vi "aal_Error Code Pool (Polynomial).vi"(1 "error":T1 items=["No Error"=0, "Err - a"=-1, "Err - b"=-2, "Warn - a"=1, "Warn - b"=2]) -> (0 "error code":i32)   [LabVIEW 2017, in "NI_AALPro.lvlib"]
uses:
  <vilib>/Analysis/NI_AALPro.lvlib
  <vilib>/Analysis/aalutilities.llb/aal_Error Code List (Polynomial).ctl
  <vilib>/Analysis/aalutilities.llb/aal_error code offset.ctl
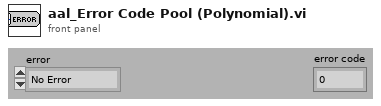
[diagram p1: front panel]
types:
  T1 = typedef "NI_AALPro.lvlib/aal_Error Code List (Polynomial).ctl" = i32
  T2 = typedef "NI_AALPro.lvlib/aal_error code offset.ctl" = i32
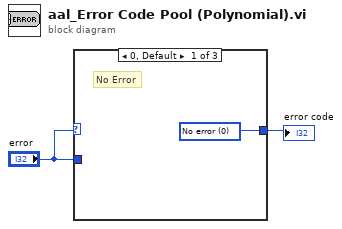
[diagram p0: block diagram]
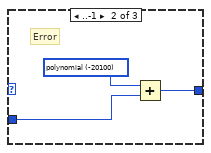
[diagram p2: hidden frame]
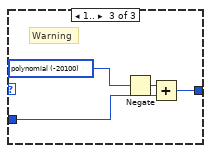
[diagram p3: hidden frame]
diagram:
  n1 = case shown="0, Default" "error" {
    tunnel: "error" -> [_ w5 w10]
    tunnel: [w3 w4 w9] -> w2
    frame 0, Default {
      w3 = 0 items=["No error", "Argument error", "Memory is full", "Out of zone", "End of file", "File already open", "Generic file I/O error", "File not found", "File permission error", "Disk is full", "Duplicate path", "Too many files open", "System feature not enabled", "Resource file not found", "Cannot add resource", "Resource not found", "Image not found", "Image memory error", "Pen does not exist", "Config type invalid", "Config token not found", "Config parse error", "Config memory error", "Bad external code format", "Bad external code offset", "External code not present", "Null window", "Destroy window error", "Null menu", "Print aborted", "Bad print record", "Print driver error", "Windows error during printing", "Memory error during printing", "Print dialog error", "Generic print error", "Invalid device refnum", "Device not found", "Device parameter error", "Device unit error", "Cannot open device", "Device call aborted", "Generic error", "Cancelled by user", "Object ID too low", "Object ID too high", "Object not in heap", "Unknown heap", "Unknown object (invalid DefProc)", "Unknown object (DefProc not in table)", "Message out of range", "Invalid (null) method", "Unknown message", "Manager call not supported", "Bad address", "Network operation in progress", "Network operation timed out", "Connection is busy", "Network attribute not supported", "Network error", "Address in use", "System out of memory", "Connection aborted", "Connection refused", "Not connected", "Already connected", "Connection closed", "Initialization error (interapplication manager)", "Bad occurrence", "Wait on unbound occurrence handler", "Occurrence queue overflow", "Datalog type conflict", "Unused", "Unrecognized type (interapplication manager)", "Memory corrupt", "Failed to make temporary DLL", "Old CIN version", "Drag socket not found", "Failed to load drop-object", "Failed to register OLE object", "Failed to release OLE object", "Format specifier type mismatch", "Unknown format specifier", "Too few format specifiers", "Too many format specifiers", "Scan failed", "Newer CIN version", "Error converting to variant", "Runtime menu error", "Password tampered", "Variant attribute not found", "Incompatible variant data type", "Event data is not available", "Event Store is not present", "Occurrence is not found", "Event Queue is not created", "Event info is not available in the type library", "Refnum passed is NULL", "Error retrieving Class GUID", "Error retrieving CoClass GUID", "Error retrieving TypeLib GUID.", "Bad built application magic bytes.", "Specific driver is different from the specific driver associated with the Logical Name.", "There is no session opened to the class driver.", "Max Error", "MAX - Error with config objects", "MAX - Error loading configuration", "MAX - Group not supported", "Singlecast connections can not send to multicast addresses.", "Multicast connections can not send to singlecast addresses.", "Specified IP address not in multicast address range.", "Attempt to write to read-only multicast connection.", "Attempt to read from write-only multicast connection.", "The buffer used to receive a datagram was smaller than the datagram itself"]
      # "No Error"
    }
    frame ..-1 {
      w6 = T2 -20100 items=["polynomial"=-20100, "special function"=-20130] ("error code offset")
      # "Error"
      n2 = Add(x=w6, y=w5) -> (x+y=w4:T2)
    }
    frame 1.. {
      w7 = T2 -20100 items=["polynomial"=-20100, "special function"=-20130, "common error"=-20000] ("error code offset")
      # "Warning"
      n3 = Negate(x=w7) -> (-x=w8:T2)
      n4 = Add(x=w8, y=w10) -> (x+y=w9:T2)
    }
  }
  "error code" <- w2
